vi "Read Log Producer.vi"(8 "error in (no error)":errorcluster, 11 "Rx Execution Unit in":refnum<class "Rx Execution Unit.lvclass">) -> (0 "error out":errorcluster, 2 "Log Producer":refnum<class "Log Producer.lvclass">, 3 "Rx Execution Unit out":refnum<class "Rx Execution Unit.lvclass">)   [LabVIEW 2020, in "Ballard ARINC 429 Engine.lvlib" / "Implementation.lvlib" / "Rx Execution Unit.lvclass"]
uses:
  Rx Execution Unit.lvclass
  Logging/Word Logging/Log Producer/Log Producer.lvclass
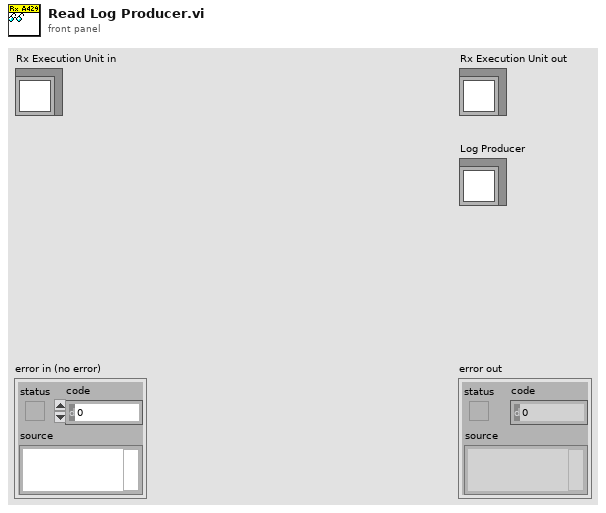
[diagram p1: front panel]
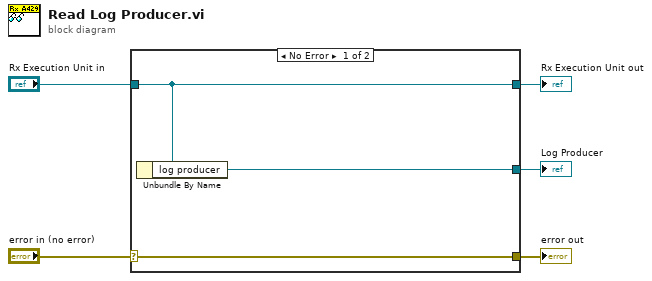
[diagram p0: block diagram]
diagram:
  n1 = case shown="No Error" "error in (no error)" {
    selector: "error in (no error)" -> [w8 w9]
    tunnel: [w8 w9] -> w4
    tunnel: [w7 w10] -> w2
    tunnel: "Rx Execution Unit in" -> [w7 w10]
    tunnel: [w6 _] -> w1
    frame No Error {
      n2 = Unbundle By Name(w7) -> ("log producer"=w6:refnum<class "Log Producer.lvclass">)
    }
    frame Error {
    }
  }
  "error out" <- w4
  "Rx Execution Unit out" <- w2
  "Log Producer" <- w1
